vi "Merge_2D_values.vi"(1 "Values In":string[][](array[string]), 2 "Present Channels":string[](array[string]), 3 "Desired Channels":string[](array[string])) -> (0 "Values Out":string[][](array[string]))   [LabVIEW 2010]
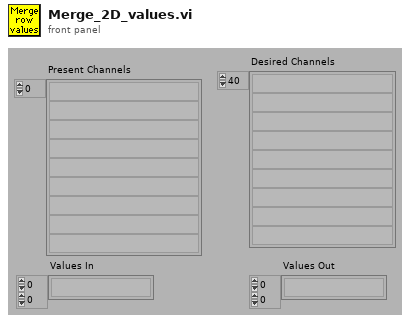
[diagram p1: front panel]
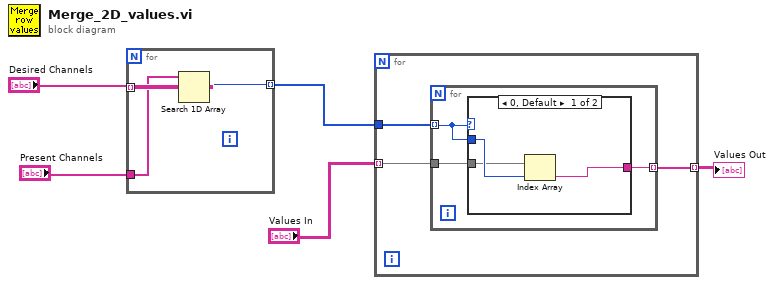
[diagram p0: block diagram]
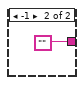
[diagram p2: hidden frame]
diagram:
  n1 = for {
    tunnel: "Present Channels" -> [w8]
    tunnel: "Desired Channels" -> [w7] mode=indexing
    tunnel: [w6] -> w3 mode=indexing
    n2 = Search 1D Array(1D array=w8, element=w7) -> (index of element=w6:i32)  [unwired: 1 out]
  }
  n3 = for {
    tunnel: w3 -> [w11]
    tunnel: "Values In" -> [w10] mode=indexing
    tunnel: [w9] -> w1 mode=indexing
    n4 = for {
      tunnel: w11 -> [w12] mode=indexing
      tunnel: w10 -> [w14]
      tunnel: [w13] -> w9 mode=indexing
      n5 = case shown="0, Default" w12 {
        tunnel: w14 -> [w15 _]
        tunnel: [w17 ""] -> w13
        tunnel: w12 -> [w16 _]
        frame 0, Default {
          n6 = Index Array(array=w15, index=w16) -> (element=w17:string)
        }
        frame -1 {
        }
      }
    }
  }
  "Values Out" <- w1
